vi "Singleton FG.vi"() -> (3 "PrefsDB":refnum<class "PrefsDB.lvclass">)   [LabVIEW 2020, in "User Prefs.lvlib" / "PrefsDB.lvclass"]
uses:
  PrefsDB.lvclass
  PrefsDB.lvclass/PrefsDB.ctl
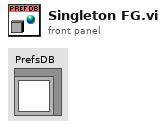
[diagram p1: front panel]
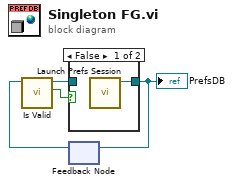
[diagram p0: block diagram]
diagram:
  n1 = feedback #1() -> (w4:refnum<class "PrefsDB.lvclass">)  [unwired: 1 in]
  n2 = call "Is Valid.vi"("PrefsDB in"=w4) -> ("Is Valid"=w3:bool, "PrefsDB out"=w2:refnum<class "PrefsDB.lvclass">)  [unwired: 8 in, 1 out]
  n3 = case shown="False" w3 {
    tunnel: w2 -> [_ w6]
    tunnel: [w5 w6] -> w1
    frame False {
      n4 = call "Launch Prefs Session.vi"() -> ("PrefsDB"=w5:refnum<class "PrefsDB.lvclass">)  [unwired: 10 in, 1 out]
    }
    frame True {
    }
  }
  "PrefsDB" <- w1
  n5 = feedback-in #1(w1) -> ()
